vi "VI Clone.vi"(8 "error in (no error)":errorcluster, 10 "Selected GObjects Only? (F)":bool, 11 "Original VI Refnum":refnum<vi>) -> (0 "error out":errorcluster, 3 "Cloned VI Refnum":refnum<vi>)   [LabVIEW 2022 SP3, in "VI-Snippet.lvlib"]
doc: "Clones the <b>Original VI Refnum</b> using VI scripting to create a new VI to avoid duplicate filenames in the same application context."
uses:
  VI-Snippet.lvlib
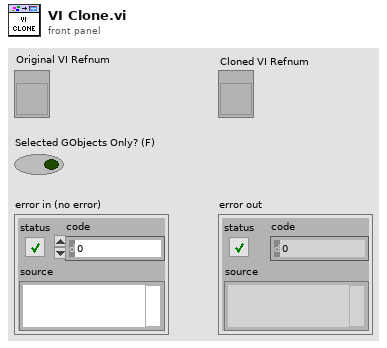
[diagram p1: front panel]
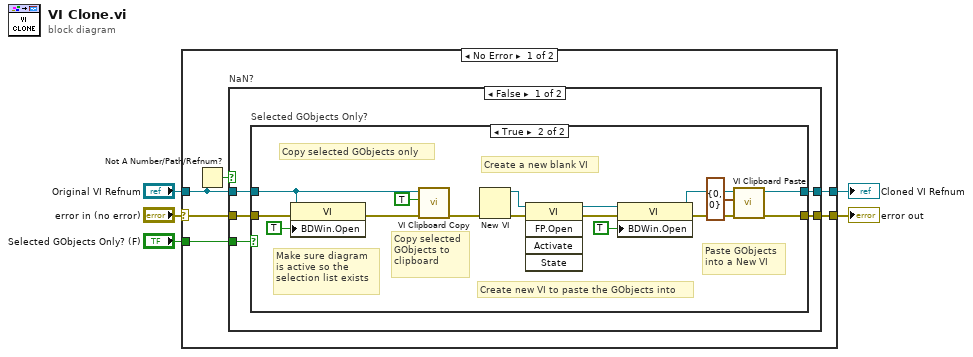
[diagram p0: block diagram]
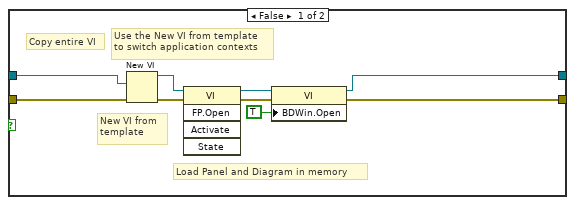
[diagram p2: hidden frame]
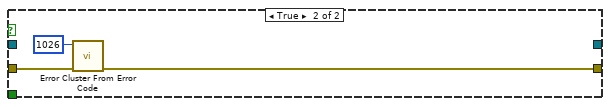
[diagram p3: hidden frame]
diagram:
  n1 = case shown="No Error" "error in (no error)" {
    selector: "error in (no error)" -> [w10 w45]
    tunnel: [w11 w45] -> w4
    tunnel: "Original VI Refnum" -> [w8 _]
    tunnel: "Selected GObjects Only? (F)" -> [w9 _]
    tunnel: [w6 _] -> w1
    frame No Error {
      n2 = Not A Number/Path/Refnum?(number/path/refnum=w8) -> (NaN/Path/Refnum?=w7:bool)
      n3 = case "NaN?" shown="False" w7 {
        tunnel: [w13 w42] -> w11
        tunnel: w10 -> [w16 w44]
        tunnel: w9 -> [w15 _]
        tunnel: w8 -> [w14 _]
        tunnel: [w12 _] -> w6
        frame False {
          n4 = case "Selected GObjects Only?" shown="True" w15 {
            tunnel: w16 -> [w25 w41]
            tunnel: w14 -> [w24 w37]
            tunnel: [w21 w40] -> w13
            tunnel: [w17 w39] -> w12
            frame False {
              # "Use the New VI from template\nto switch application contexts"
              # "Load Panel and Diagram in memory"
              # "New VI from\ntemplate"
              # "Copy entire VI"
              n5 = New VI(8:w25, 10:w24) -> (0:w23:errorcluster, 3:w18:refnum<vi>)  [unwired: 5 in]
              n6 = invoke class="VI" method="FP.Open"(reference=w18, error in=w23) -> (reference out=w20:refnum<vi>, error out=w22:errorcluster)  [unwired: 3 in, 3 out]
              n7 = property class="VI"(reference=w20, error in=w22, "BDWin.Open"=TRUE ("Block Diagram Window:Open")) -> (reference out=w17:refnum<vi>, error out=w21:errorcluster)
            }
            frame True {
              # "Create a new blank VI"
              # "Make sure diagram\nis active so the\nselection list exists"
              # "Create new VI to paste the GObjects into"
              # "Paste GObjects\ninto a New VI"
              # "Copy selected\nGObjects to\nclipboard"
              # "Copy selected GObjects only"
              n8 = property class="VI"(reference=w37, error in=w41, "BDWin.Open"=TRUE ("Block Diagram Window:Open")) -> (error out=w38:errorcluster)  [unwired: 1 out]
              n9 = call "VI Clipboard Copy.vi"("error in (no error)"=w38, "Selection List Only? (F=All)"=TRUE ("Selected GObjects Only? (F)"), "VI Refnum in"=w37) -> ("error out"=w30:errorcluster)  [unwired: 7 in, 1 out]
              n10 = New VI(8:w30) -> (0:w35:errorcluster, 3:w34:refnum<vi>)  [unwired: 6 in]
              n11 = invoke class="VI" method="FP.Open"(reference=w34, error in=w35) -> (reference out=w33:refnum<vi>, error out=w32:errorcluster)  [unwired: 3 in, 3 out]
              n12 = property class="VI"(reference=w33, error in=w32, "BDWin.Open"=TRUE ("Block Diagram Window:Open")) -> (reference out=w28:refnum<vi>, error out=w29:errorcluster)
              n13 = call "VI Clipboard Paste.vi"("error in (no error)"=w29, "Drop Position (0, 0)"=cluster{"Left":i32, "Top":i32} {"Left"=0, "Top"=0}, "VI Refnum in"=w28) -> ("error out"=w40:errorcluster, "VI Refnum out"=w39:refnum<vi>)  [unwired: 7 in]
            }
          }
        }
        frame True {
          n14 = call <vilib>:"Error Cluster From Error Code.vi"("error in (no error)"=w44, "error code (0)"=1026) -> ("error out"=w42:errorcluster)  [unwired: 7 in]
        }
      }
    }
    frame Error {
    }
  }
  "error out" <- w4
  "Cloned VI Refnum" <- w1
